vi "Enable Power Control.vi"(7 "Address (1)":u16=1 max=15 step=1, 8 "error in (no error)":errorcluster, 9 "Enable Valve Motor Power (Disable)":bool, 10 "Enable Syringe Motor Power (Disable)":bool, 11 "VISA resource name":refnum<visa-resource-name>) -> (0 "error out":errorcluster, 3 "VISA resource name out":refnum<visa-resource-name>)   [LabVIEW 2021, in "Copy of Kloehn V6 Series.lvlib"]
doc: "Enables power control over the syringe and valve motor . Since at times, the syringe motor can be turned half on, it can be valuable to be able to turn it off because it can be loud."
uses:
  Copy of Kloehn V6 Series.lvlib
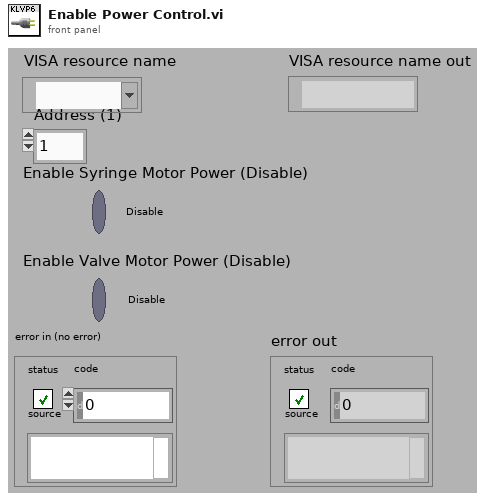
[diagram p1: front panel]
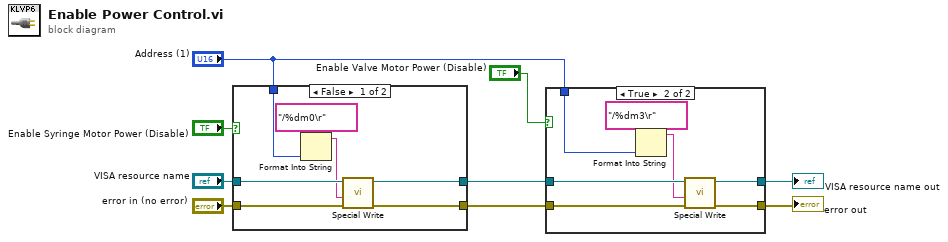
[diagram p0: block diagram]
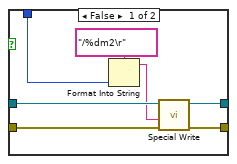
[diagram p2: hidden frame]
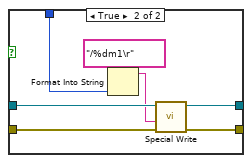
[diagram p3: hidden frame]
diagram:
  n1 = case shown="False" "Enable Syringe Motor Power (Disable)" {
    tunnel: "error in (no error)" -> [w16 w21]
    tunnel: [w15 w20] -> w6
    tunnel: "VISA resource name" -> [w14 w22]
    tunnel: [w13 w23] -> w5
    tunnel: "Address (1)" -> [w11 w18]
    frame False {
      n2 = Format Into String(format string="/%dm0\r" ("Send String"), w11) -> (resulting string=w10:string)  [unwired: 2 in, 1 out]
      n3 = call "Special Write.vi"("error in (no error)"=w16, "Send String"=w10, "VISA resource name"=w14) -> ("error out"=w15:errorcluster, "VISA resource name out"=w13:refnum<visa-resource-name>)  [unwired: 4 in, 3 out]
    }
    frame True {
      n4 = Format Into String(format string="/%dm1\r" ("Send String"), w18) -> (resulting string=w17:string)  [unwired: 2 in, 1 out]
      n5 = call "Special Write.vi"("error in (no error)"=w21, "Send String"=w17, "VISA resource name"=w22) -> ("error out"=w20:errorcluster, "VISA resource name out"=w23:refnum<visa-resource-name>)  [unwired: 4 in, 3 out]
    }
  }
  n6 = case shown="True" "Enable Valve Motor Power (Disable)" {
    tunnel: w6 -> [w29 w37]
    tunnel: [w28 w36] -> w4
    tunnel: [w27 w35] -> w2
    tunnel: w5 -> [w30 w34]
    tunnel: "Address (1)" -> [w25 w32]
    frame False {
      n7 = Format Into String(format string="/%dm2\r" ("Send String"), w25) -> (resulting string=w24:string)  [unwired: 2 in, 1 out]
      n8 = call "Special Write.vi"("error in (no error)"=w29, "Send String"=w24, "VISA resource name"=w30) -> ("error out"=w28:errorcluster, "VISA resource name out"=w27:refnum<visa-resource-name>)  [unwired: 4 in, 3 out]
    }
    frame True {
      n9 = Format Into String(format string="/%dm3\r" ("Send String"), w32) -> (resulting string=w31:string)  [unwired: 2 in, 1 out]
      n10 = call "Special Write.vi"("error in (no error)"=w37, "Send String"=w31, "VISA resource name"=w34) -> ("error out"=w36:errorcluster, "VISA resource name out"=w35:refnum<visa-resource-name>)  [unwired: 4 in, 3 out]
    }
  }
  "error out" <- w4
  "VISA resource name out" <- w2
